vi "Launch child actors.vi"(8 "error in (no error)":errorcluster, 11 "Controller in":refnum<class "Controller.lvclass">) -> (0 "error out":errorcluster, 3 "Controller out":refnum<class "Controller.lvclass">)   [LabVIEW 2011, in "Controller.lvclass"]
uses:
  Controller.lvclass
  UI/Remote/Remote UI.lvclass
  DAQ/DAQ.lvclass
  <userlib>/_Frameworks/ActorFramework/Actor/Actor.lvclass/Actor.ctl
  <userlib>/_Frameworks/ActorFramework/Message Enqueuer/Message Enqueuer.lvclass/Message Enqueuer.ctl
  Controller.lvclass/Controller.ctl
  <userlib>/_Frameworks/ActorFramework/Message Enqueuer/Init from Existing Queue.vi
  <userlib>/_Frameworks/ActorFramework/Message Enqueuer/Message Enqueuer.lvclass
  <userlib>/_Frameworks/ActorFramework/Actor/Actor.lvclass
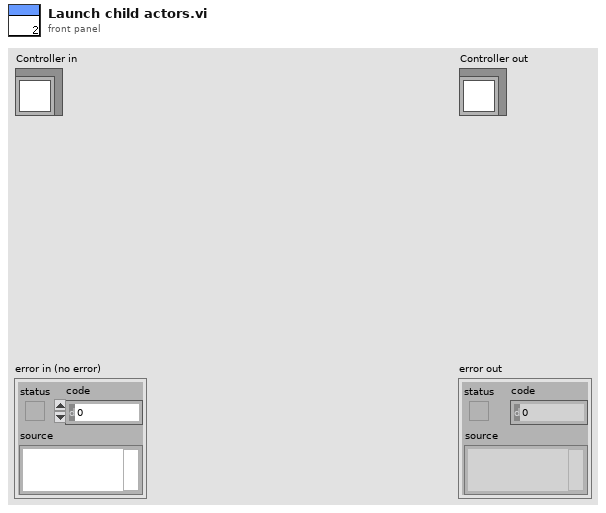
[diagram p1: front panel]
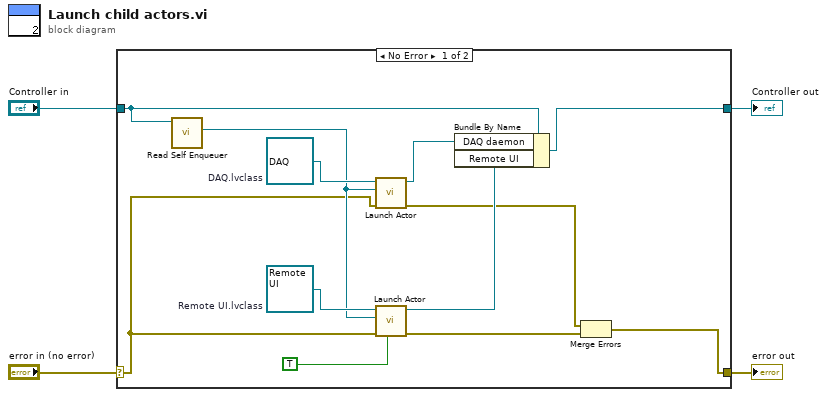
[diagram p0: block diagram]
diagram:
  n1 = case shown="No Error" "error in (no error)" {
    selector: "error in (no error)" -> [w9 w18]
    tunnel: [w8 w18] -> w3
    tunnel: [w6 w17] -> w1
    tunnel: "Controller in" -> [w7 w17]
    frame No Error {
      w15 = refnum<class "Remote UI.lvclass"> refnum  # Remote UI.lvclass
      w16 = refnum<class "DAQ.lvclass"> refnum  # DAQ.lvclass
      n2 = call <userlib>:"Read Self Enqueuer.vi"("Actor"=w7) -> ("Self Enqueuer"=w14:refnum<class "Message Enqueuer.lvclass">)  [unwired: 10 in]
      n3 = call <userlib>:"Launch Actor.vi"("error in (no error)"=w9, "Actor-to-Caller Enqueuer"=w14, "Actor"=w16) -> ("error out"=w11:errorcluster, "Caller-To-Actor Enqueuer"=w13:refnum<class "Message Enqueuer.lvclass">)  [unwired: 7 in]
      n4 = call <userlib>:"Launch Actor.vi"("Open Actor Core front panel? (F)"=TRUE, "error in (no error)"=w9, "Actor-to-Caller Enqueuer"=w14, "Actor"=w15) -> ("error out"=w5:errorcluster, "Caller-To-Actor Enqueuer"=w12:refnum<class "Message Enqueuer.lvclass">)  [unwired: 6 in]
      n5 = Bundle By Name(cluster=w7, "DAQ daemon"=w13, "Remote UI"=w12) -> (w6:refnum<class "Controller.lvclass">)
      n6 = Merge Errors(w11, w5) -> (w8:errorcluster)
    }
    frame Error {
    }
  }
  "error out" <- w3
  "Controller out" <- w1
